vi "Check Gate Calculation Type.vi"(8 "Error In":errorcluster, 10 "Gates Definitions in":T1={"First Gate: t1"=0.0, "Gate Width: W"=0.0, "Gate Step: d"=0.0, "# Gates: G"=0.0, "Use Gate Center"=FALSE, "Frames/Image: F"=0, "Gates/Frame: L"=0, "Bits/Frame: q"=0, "Multiplicity: p"=0, "Gate Type"=enum."Square", "Gate Edge s"=0.0, "Gate Top Slope"=0.0, "Reversed Sawtooth?"=FALSE, "Computation"=FALSE, "User-defined Gate"={"X Array"=[], "Y Array"=[]}, "Tolerance"=0.0, "Integration"=enum."Item 0", "# Steps"=50.0, "Type of User-defined Function"=enum."Gate"}, 11 "Phasor Calculation Type in":T4) -> (0 "Error Out":errorcluster, 2 "Gates Definitions out":T1={"First Gate: t1"=0.0, "Gate Width: W"=0.0, "Gate Step: d"=0.0, "# Gates: G"=0.0, "Use Gate Center"=FALSE, "Frames/Image: F"=0, "Gates/Frame: L"=0, "Bits/Frame: q"=0, "Multiplicity: p"=0, "Gate Type"=enum."Square", "Gate Edge s"=0.0, "Gate Top Slope"=0.0, "Reversed Sawtooth?"=FALSE, "Computation"=FALSE, "User-defined Gate"={"X Array"=[], "Y Array"=[]}, "Tolerance"=0.0, "Integration"=enum."Item 0", "# Steps"=50.0, "Type of User-defined Function"=enum."Gate"}, 3 "Phasor Calculation Type out":T4)   [LabVIEW 2019]
uses:
  Phasor Calculation Type.ctl
  Gate Definitions.ctl
  Gate Type.ctl
  Graphs/XY Graph/XY Plot Data.ctl
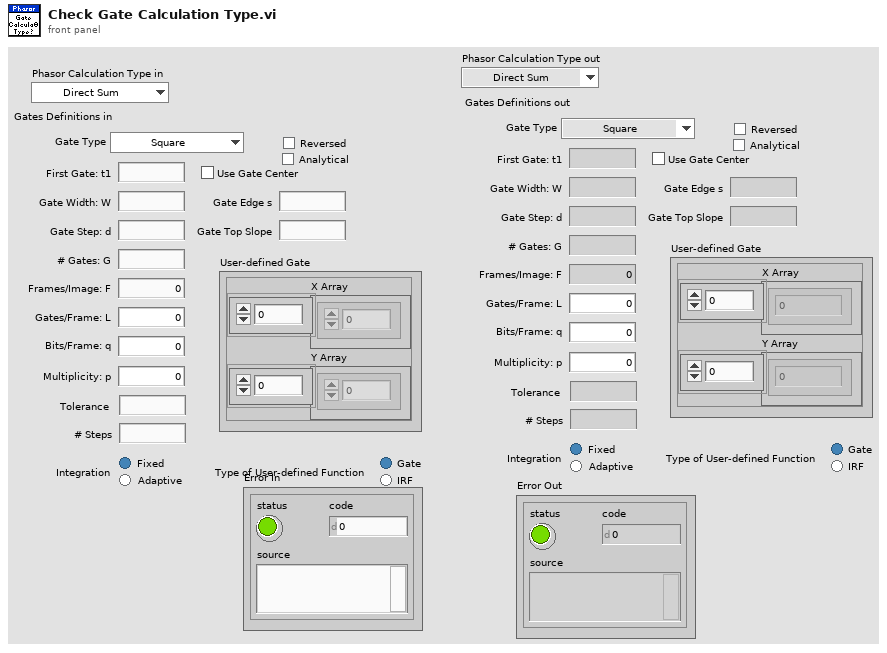
[diagram p1: front panel]
types:
  T1 = typedef "Gate Definitions.ctl" = cluster{"First Gate: t1":ext, "Gate Width: W":ext, "Gate Step: d":ext, "# Gates: G":ext, "Use Gate Center":bool, "Frames/Image: F":i32, "Gates/Frame: L":i32, "Bits/Frame: q":i32, "Multiplicity: p":i32, "Gate Type":T2, "Gate Edge s":ext, "Gate Top Slope":ext, "Reversed Sawtooth?":bool, "Computation":bool, "User-defined Gate":T3, "Tolerance":ext, "Integration":enum32{"Item 0", "Item 1"}, "# Steps":ext, "Type of User-defined Function":enum32{"Gate", "IRF"}}
  T2 = typedef "Gate Type.ctl" = enum16{"Square", "Finite Edge Square", "Finite Edge, Tilted Top Square", "Triangle", "Sawtooth", "User-defined"}
  T3 = typedef "XY Plot Data.ctl" = cluster{"X Array":dbl[], "Y Array":dbl[]}
  T4 = typedef "Phasor Calculation Type.ctl" = enum16{"Direct Sum", "Analytical Formula"}
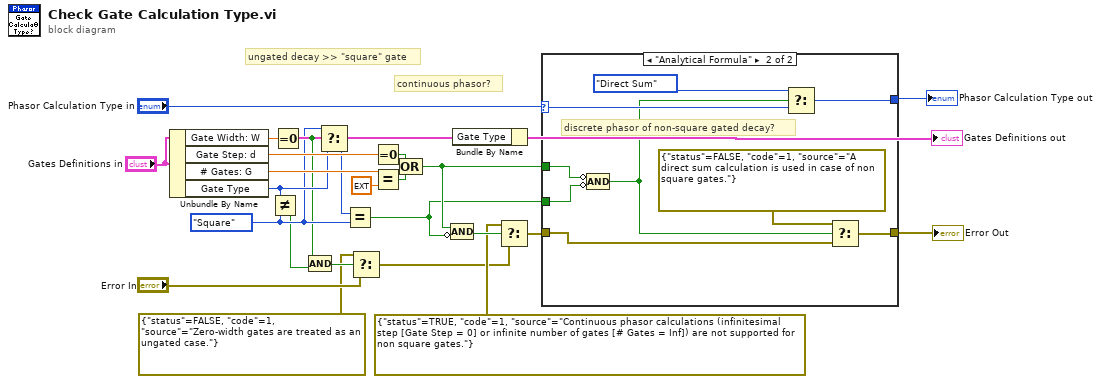
[diagram p0: block diagram]
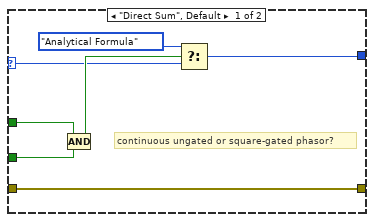
[diagram p2: hidden frame]
diagram:
  w7 = Gate_Type."Square" ("y")
  # "ungated decay >> \"square\" gate"
  # "continuous phasor?"
  n1 = Unbundle By Name("Gates Definitions in") -> ("Gate Width: W"=w12:ext, "Gate Step: d"=w22:ext, "# Gates: G"=w20:ext, "Gate Type"=w8:T2)
  n2 = Not Equal?(x=w8, y=w7) -> (x != y?=w5:bool)
  n3 = Equal To 0?(x=w12) -> (x = 0?=w6:bool)
  n4 = Compound Arithmetic op=AND(w6, w5) -> (w4:bool)
  n5 = Select(t=w7, s=w6, f=w8) -> (s? t:f=w10:T2)
  n6 = Equal?(x=w10, y=w7) -> (x = y?=w16:bool)
  n7 = Select(t=errorcluster {"status"=FALSE, "code"=1, "source"="Zero-width gates are treated as an ungated case."}, s=w4, f="Error In") -> (s? t:f=w2:errorcluster)
  n8 = Equal To 0?(x=w22) -> (x = 0?=w19:bool)
  n9 = Equal?(x=w20, y=ext inf) -> (x = y?=w18:bool)
  n10 = Compound Arithmetic op=OR(w19, w18) -> (w17:bool)
  n11 = Compound Arithmetic op=AND(w17, invert w16) -> (w15:bool)
  n12 = Bundle By Name(cluster="Gates Definitions in", "Gate Type"=w10) -> (→"Gates Definitions out":T1)
  n13 = Select(t=errorcluster {"status"=TRUE, "code"=1, "source"="Continuous phasor calculations (infinitesimal step [Gate Step = 0] or infinite number of gates [# Gates = Inf]) are not supported for non square gates."}, s=w15, f=w2) -> (s? t:f=w13:errorcluster)
  n14 = case shown="\"Analytical Formula\"" "Phasor Calculation Type in" {
    selector: "Phasor Calculation Type in" -> [w29 w39]
    tunnel: [w31 w41] -> w25
    tunnel: [w26 w37] -> w23
    tunnel: w16 -> [w28 w36]
    tunnel: w17 -> [w27 w35]
    tunnel: w13 -> [w26 w33]
    frame "Direct Sum", Default {
      # "continuous ungated or square-gated phasor?"
      n15 = Compound Arithmetic op=AND(w27, w28) -> (w32:bool)
      n16 = Select(t=Phasor_Calculation_Type."Analytical Formula", s=w32, f=w29) -> (s? t:f=w31:T4)
    }
    frame "Analytical Formula" {
      # "discrete phasor of non-square gated decay?"
      n17 = Compound Arithmetic op=AND(invert w35, invert w36) -> (w38:bool)
      n18 = Select(t=Phasor_Calculation_Type."Direct Sum", s=w38, f=w39) -> (s? t:f=w41:T4)
      n19 = Select(t=errorcluster {"status"=FALSE, "code"=1, "source"="A direct sum calculation is used in case of non square gates."}, s=w38, f=w33) -> (s? t:f=w37:errorcluster)
    }
  }
  "Phasor Calculation Type out" <- w25
  "Error Out" <- w23
